vi "华为UPS2000-G获取电池状态.vi"(8 "error in (no error)":errorcluster, 11 "MB session in":refnum<class "MB_Master.lvclass">) -> (0 "error out":errorcluster, 2 "电池状态":T1 {"电池状态" items=["休眠"=2, "浮充"=3, "均充"=4, "放电"=5]}, 3 "MB session out":refnum<class "MB_Master.lvclass">)   [LabVIEW 2016, in "环境动力监测库.lvlib" / "UPS库.lvlib"]
uses:
  <vilib>/Plasmionique/MB Master/MB_Master/MB_Master.lvclass
  <vilib>/Plasmionique/MB Master/MB Master.lvlib
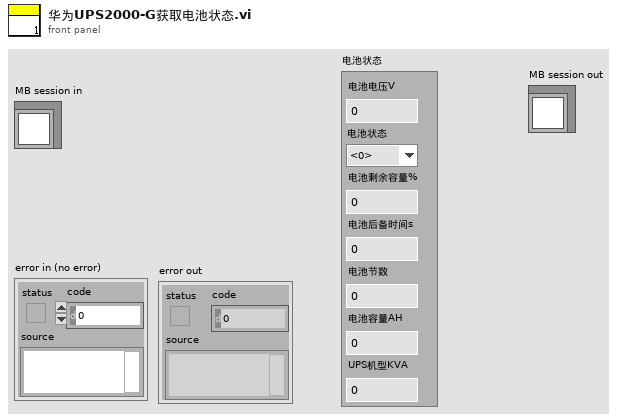
[diagram p1: front panel]
types:
  T1 = cluster{"电池电压V":dbl, "电池状态":u16, "电池剩余容量%":u16, "电池后备时间s":u32, "电池节数":u16, "电池容量AH":u16, "UPS机型KVA":u16}
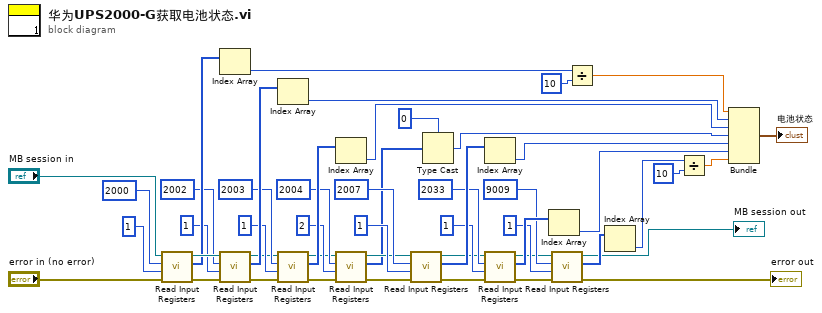
[diagram p0: block diagram]
diagram:
  n1 = call <vilib>:"Read Input Registers.vi"("error in (no error)"="error in (no error)", "quantity"=u16 1, "starting address"=u16 2000, "MB session in"="MB session in") -> ("error out"=w39:errorcluster, "Registers"=w45:u16[], "MB session out"=w48:refnum<class "MB_Master.lvclass">)  [unwired: 5 in]
  n2 = Index Array(array=w45) -> (element=w43:u16)  [unwired: 1 in]
  n3 = call <vilib>:"Read Input Registers.vi"("error in (no error)"=w39, "quantity"=u16 1, "starting address"=u16 2002, "MB session in"=w48) -> ("error out"=w34:errorcluster, "Registers"=w38:u16[], "MB session out"=w35:refnum<class "MB_Master.lvclass">)  [unwired: 5 in]
  n4 = Index Array(array=w38) -> (element=w12:u16)  [unwired: 1 in]
  n5 = call <vilib>:"Read Input Registers.vi"("error in (no error)"=w34, "quantity"=u16 1, "starting address"=u16 2003, "MB session in"=w35) -> ("error out"=w29:errorcluster, "Registers"=w33:u16[], "MB session out"=w30:refnum<class "MB_Master.lvclass">)  [unwired: 5 in]
  n6 = Index Array(array=w33) -> (element=w11:u16)  [unwired: 1 in]
  n7 = call <vilib>:"Read Input Registers.vi"("error in (no error)"=w29, "quantity"=u16 2, "starting address"=u16 2004, "MB session in"=w30) -> ("error out"=w25:errorcluster, "Registers"=w9:u16[], "MB session out"=w26:refnum<class "MB_Master.lvclass">)  [unwired: 5 in]
  n8 = call <vilib>:"Read Input Registers.vi"("error in (no error)"=w25, "quantity"=u16 1, "starting address"=u16 2007, "MB session in"=w26) -> ("error out"=w20:errorcluster, "Registers"=w24:u16[], "MB session out"=w21:refnum<class "MB_Master.lvclass">)  [unwired: 5 in]
  n9 = Type Cast(type=u32 0, x=w9) -> (*(type *) &x=w8:u32)
  n10 = Index Array(array=w24) -> (element=w7:u16)  [unwired: 1 in]
  n11 = call <vilib>:"Read Input Registers.vi"("error in (no error)"=w20, "quantity"=u16 1, "starting address"=u16 2033, "MB session in"=w21) -> ("error out"=w15:errorcluster, "Registers"=w19:u16[], "MB session out"=w16:refnum<class "MB_Master.lvclass">)  [unwired: 5 in]
  n12 = Index Array(array=w19) -> (element=w6:u16)  [unwired: 1 in]
  n13 = call <vilib>:"Read Input Registers.vi"("error in (no error)"=w15, "quantity"=u16 1, "starting address"=u16 9009, "MB session in"=w16) -> ("error out"=→"error out":errorcluster, "Registers"=w14:u16[], "MB session out"=→"MB session out":refnum<class "MB_Master.lvclass">)  [unwired: 5 in]
  n14 = Divide(x=w43, y=u16 10) -> (x/y=w42:dbl)
  n15 = Index Array(array=w14) -> (element=w4:u16)  [unwired: 1 in]
  n16 = Divide(x=w4, y=u16 10) -> (x/y=w3:dbl)
  n17 = Bundle(w42, w12, w11, w8, w7, w6, w3) -> (→"电池状态":cluster{dbl, u16, u16, u32, u16, u16, dbl})  [unwired: 1 in]
